vi "Actor Launched.vi"(6 "Actor Type":string, 7 "Actor Core VI":string, 8 "error in (no error)":errorcluster, 9 "Actor's Caller Q":refnum<class "Message Enqueuer.lvclass">, 10 "Actor's Self Q":refnum<class "Message Enqueuer.lvclass">, 11 "Actor Monitor New in":refnum<class "Actor Monitor.lvclass">) -> (0 "error out":errorcluster, 3 "Actor Monitor New out":refnum<class "Actor Monitor.lvclass">)   [LabVIEW 2020, in "Monitored Actor.lvlib" / "Actor Monitor.lvclass"]
doc: "Adds the new actor to the monitored data object\n\nCopyright: MGI 2016\nAuthor: Derek Trepanier"
uses:
  <vilib>/MGI/Monitored Actor/Actor Monitor/Actor Monitor/Actor Monitor.lvclass
  <vilib>/ActorFramework/Message Enqueuer/Message Enqueuer.lvclass
  <vilib>/MGI/Monitored Actor/Actor Monitor/Actor Monitor/Actor Monitor.lvclass/Actor Monitor.ctl
  <vilib>/MGI/Monitored Actor/Monitor Data/Monitor Data.lvclass
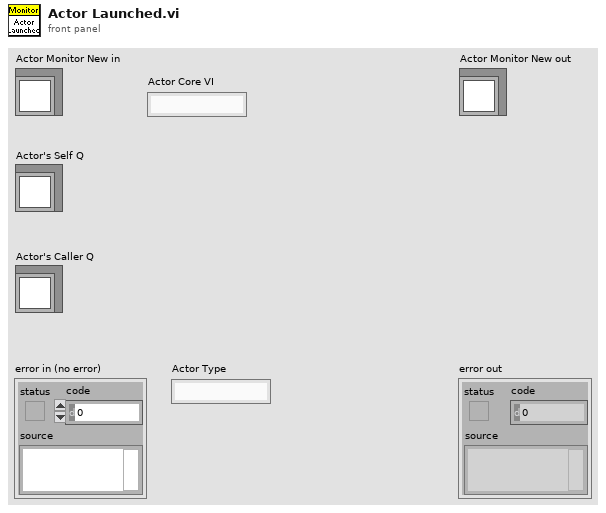
[diagram p1: front panel]
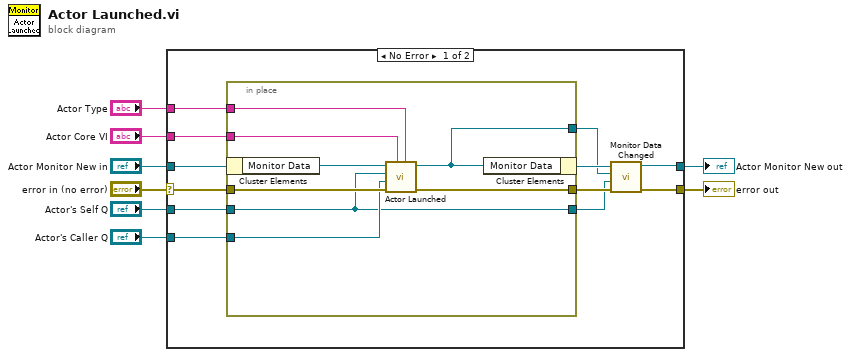
[diagram p0: block diagram]
diagram:
  n1 = case shown="No Error" "error in (no error)" {
    selector: "error in (no error)" -> [w18 w30]
    tunnel: [w14 w30] -> w7
    tunnel: [w12 w29] -> w5
    tunnel: "Actor Monitor New in" -> [w20 w29]
    tunnel: "Actor Core VI" -> [w17 _]
    tunnel: "Actor's Self Q" -> [w16 _]
    tunnel: "Actor's Caller Q" -> [w15 _]
    tunnel: "Actor Type" -> [w9 _]
    frame No Error {
      n2 = in-place {
        in-place-border: [w27] -> w19
        in-place-border: w18 -> [w26]
        in-place-border: w17 -> [w25]
        in-place-border: w16 -> [w22]
        in-place-border: w15 -> [w24]
        in-place-border: [w23] -> w11
        in-place-border: [w22] -> w10
        in-place-border: w9 -> [w21]
        n3 = in-place-cluster #1(w20) -> ("Monitor Data"=w28:refnum<class "Monitor Data.lvclass">)
        n4 = call <vilib>:"Actor Launched.vi"("Actor Type"=w21, "Actor Core VI"=w25, "error in (no error)"=w26, "Actor's Caller Q"=w24, "Actor's Self Q"=w22, "Monitor Data in"=w28) -> ("error out"=w27:errorcluster, "Monitor Data out"=w23:refnum<class "Monitor Data.lvclass">)  [unwired: 4 in]
        n5 = in-place-cluster #1("Monitor Data"=w23) -> (w13:refnum<class "Actor Monitor.lvclass">)
      }
      n6 = call-dynamic "Monitor Data Changed.vi"("error in (no error)"=w19, "Changed Actor's Q"=w10, "Monitor Data"=w11, "Actor Monitor New in"=w13) -> ("error out"=w14:errorcluster, "Actor Monitor New out"=w12:refnum<class "Actor Monitor.lvclass">)  [unwired: 6 in]
    }
    frame Error {
    }
  }
  "error out" <- w7
  "Actor Monitor New out" <- w5
